vi "Edit TCP Ports.vi"(8 "error in":errorcluster) -> (0 "error out":errorcluster)   [LabVIEW 2024, in "User Interface.lvlib"]
uses:
  User Interface.lvlib
  Support/General Type Defs/Edit Devices States.ctl
  <vilib>/Utility/miscctls.llb/LVRowAndColumnTypeDef.ctl
  <vilib>/Utility/error.llb/Trim Whitespace One-Sided.vi
  Support/General Type Defs/Global Data.vi
  Data Base/DataBase Queue - Enqueue.vi
  Support/General Type Defs/General Type Definitions.lvlib
  Data Base/Data Base.lvlib
panel:
  out "Port To Delete":string[](array[string])
  in  "Delete":bool
  in  "Linux TCP Ports":string[][](table)
  in  "Windows TCP Ports":string[][](table)
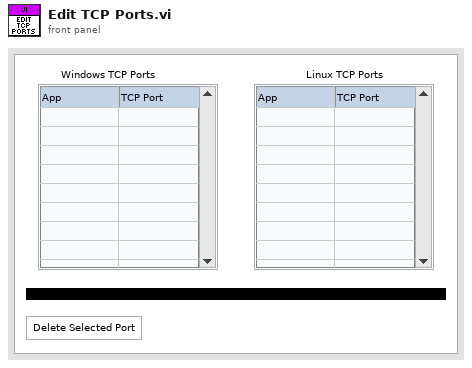
[diagram p1: front panel]
types:
  T1 = typedef "General Type Definitions.lvlib/Edit Devices States.ctl" = enum16{"Init", "IDLE", "Display Selection", "Clean Selection", "Delete", "Update", "Save Changes", "STOP"}
  T2 = typedef "LVRowAndColumnTypeDef.ctl" = cluster{"Row":i32, "Column":i32}
  T3 = enum16{"Left Button", "Center Button", "Right Button", "Window Close"}
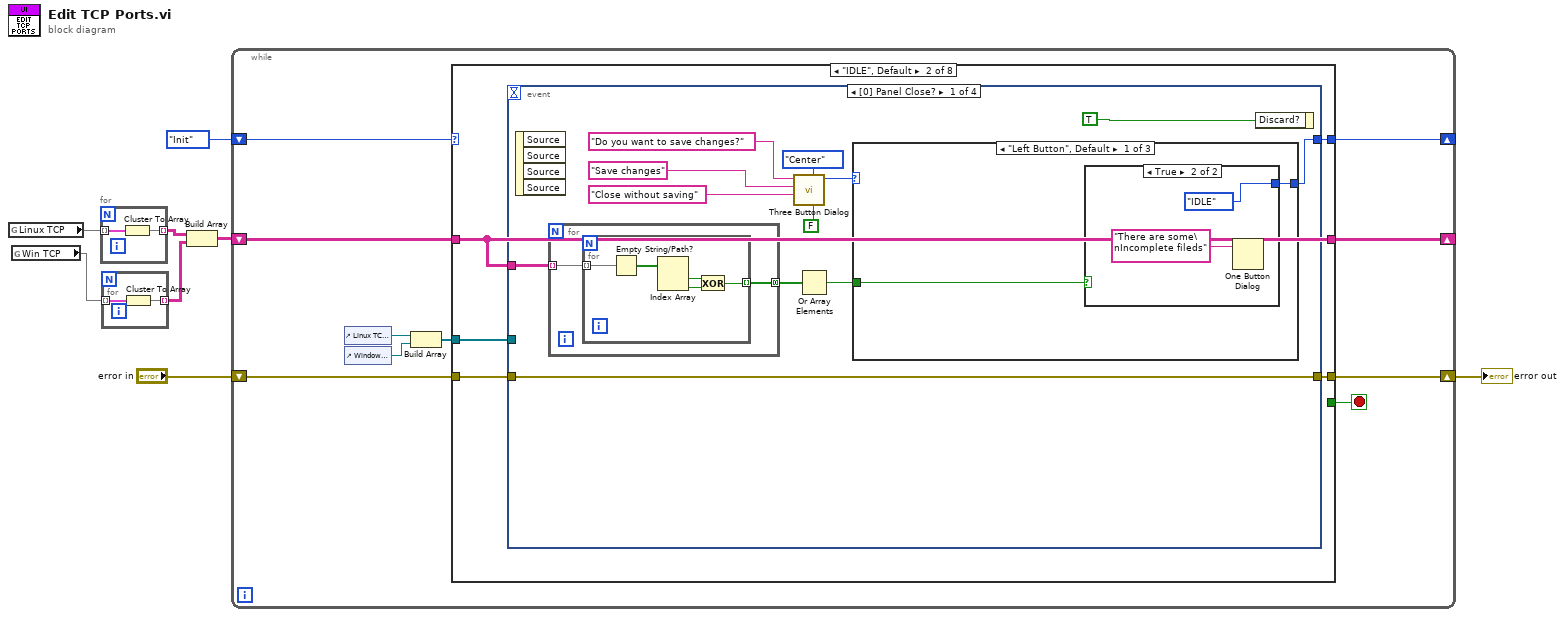
[diagram p0: block diagram]
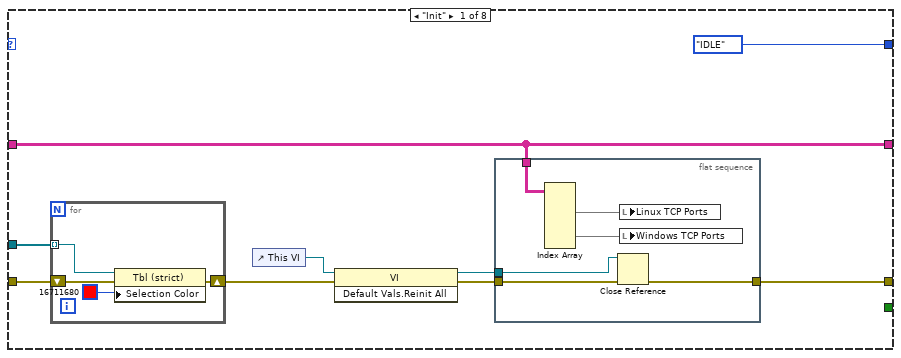
[diagram p2: hidden frame]
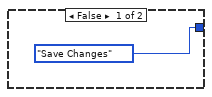
[diagram p3: hidden frame]
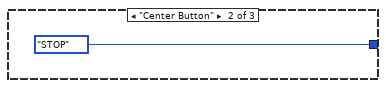
[diagram p4: hidden frame]
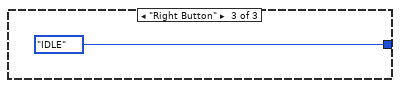
[diagram p5: hidden frame]
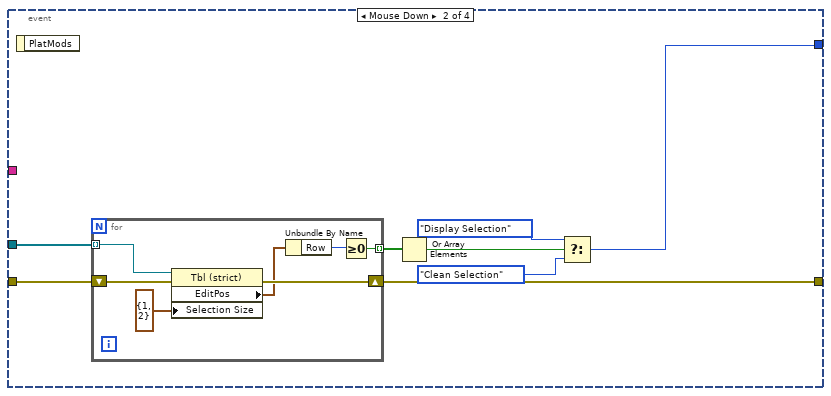
[diagram p6: hidden frame]
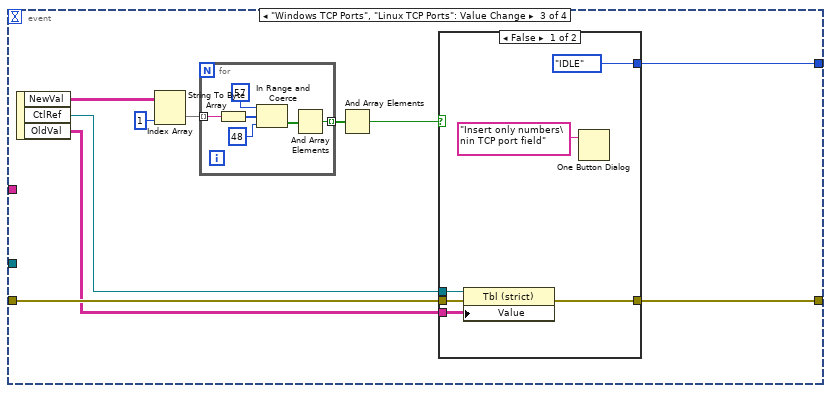
[diagram p7: hidden frame]
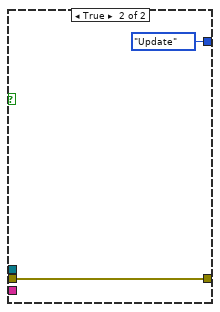
[diagram p8: hidden frame]
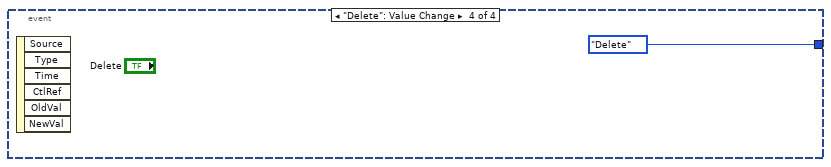
[diagram p9: hidden frame]
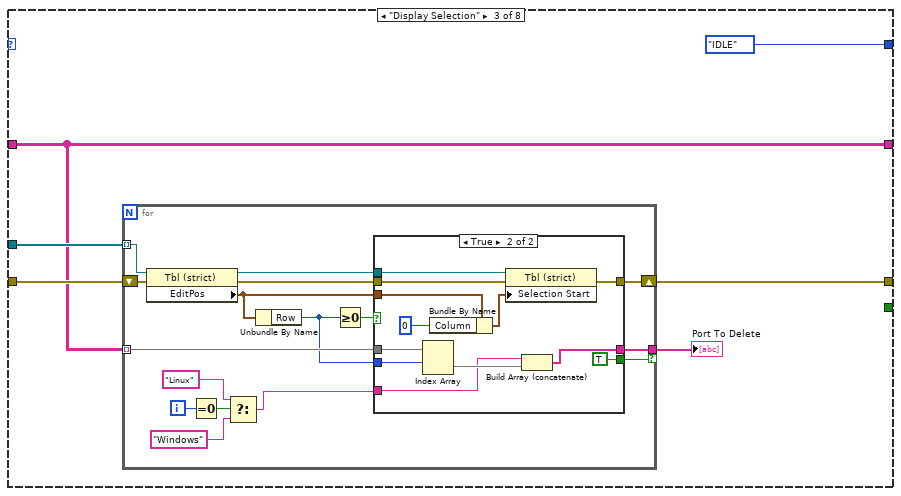
[diagram p10: hidden frame]
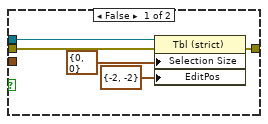
[diagram p11: hidden frame]
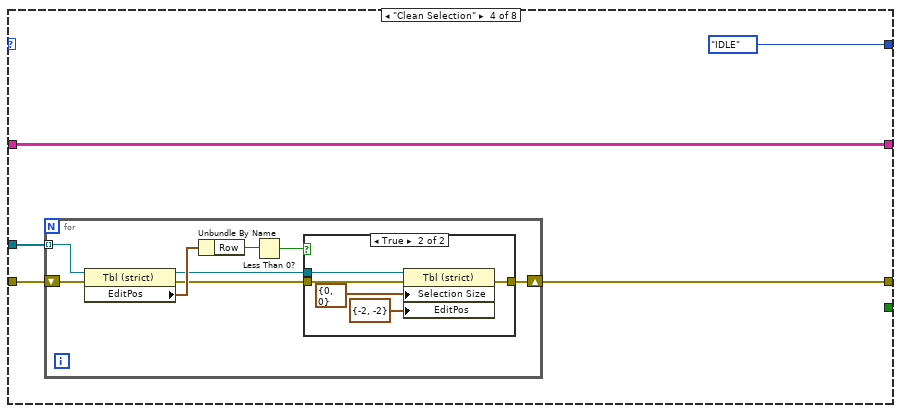
[diagram p12: hidden frame]
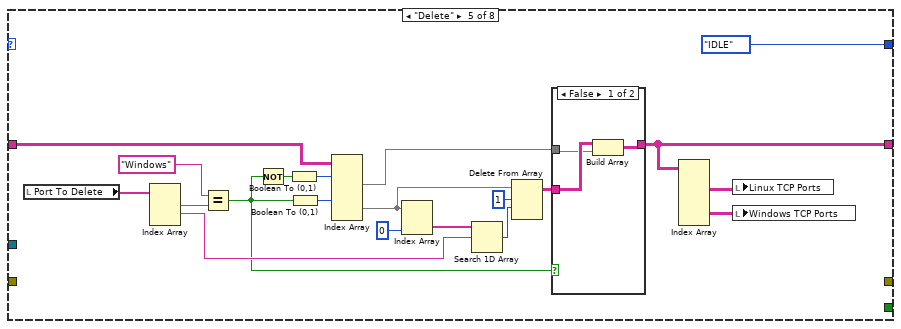
[diagram p14: hidden frame]
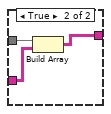
[diagram p15: hidden frame]
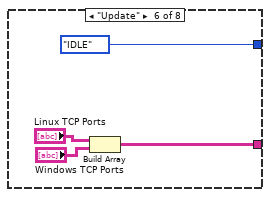
[diagram p16: hidden frame]
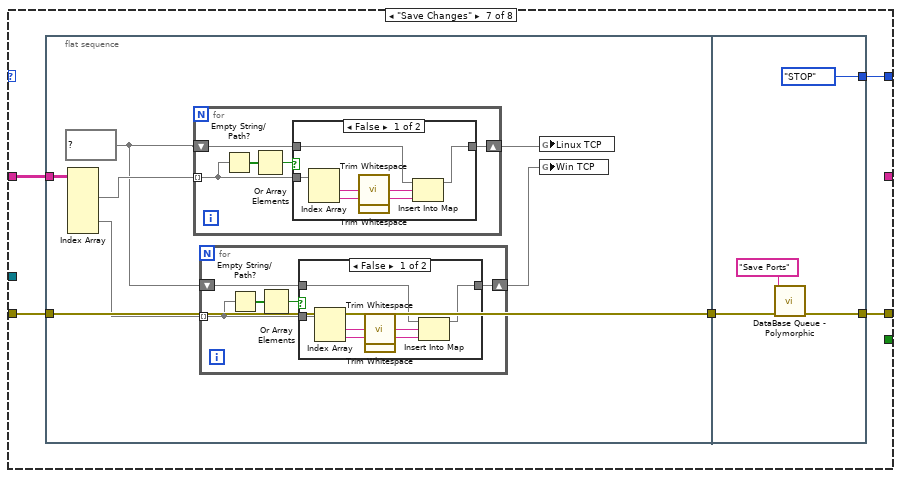
[diagram p17: hidden frame]
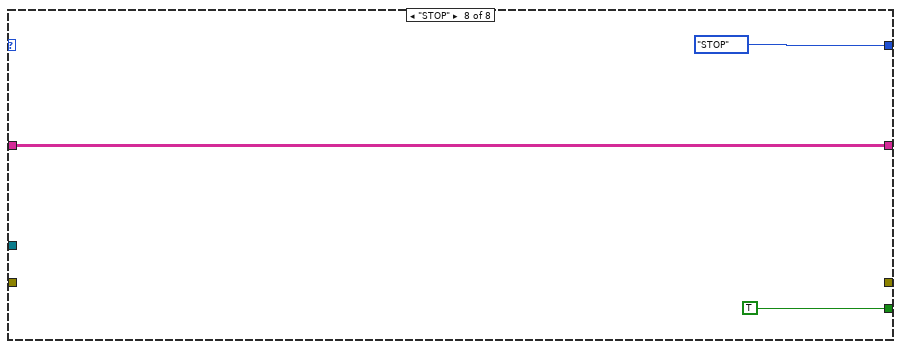
[diagram p20: hidden frame]
diagram:
  n1 = global read "Global Data.vi" "Linux TCP"() -> (w7:map{string, string})
  n2 = global read "Global Data.vi" "Win TCP"() -> (w2:map{string, string})
  n3 = for {
    tunnel: w7 -> [w10] mode=indexing
    tunnel: [w9] -> w5 mode=indexing
    n4 = Cluster To Array(cluster=w10) -> (array=w9:string[])
  }
  n5 = for {
    tunnel: [w12] -> w1 mode=indexing
    tunnel: w2 -> [w11] mode=indexing
    n6 = Cluster To Array(cluster=w11) -> (array=w12:string[])
  }
  n7 = Build Array(w5, w1) -> (w4:string[][][])
  n8 = while {
    shift-right: [w21] -> _
    shift-left: Edit_Devices_States."Init" ("Enum") -> [w22]
    shift-right: [w13] -> _
    shift-left: w4 -> [w16]
    shift-right: [w18] -> w3
    shift-left: "error in" -> [w19]
    stop <- w20 stop-if-true
    n9 = control-ref of="Linux TCP Ports"() -> (w15:refnum<vi>)
    n10 = control-ref of="Windows TCP Ports"() -> (w14:refnum<vi>)
    n11 = Build Array(w15, w14) -> (w17:refnum<vi>[])
    n12 = case shown="\"IDLE\", Default" w22 {
      tunnel: w16 -> [w23 w42 w114 w156 w183 _ w205 w245]
      tunnel: [w23 w42 w114 w156 w173 w198 _ w245] -> w13
      tunnel: [Edit_Devices_States."IDLE" ("Enum") w46 Edit_Devices_States."IDLE" Edit_Devices_States."IDLE" Edit_Devices_States."IDLE" Edit_Devices_States."IDLE" w201 Edit_Devices_States."STOP"] -> w21
      tunnel: [_ _ _ _ _ _ _ TRUE] -> w20
      tunnel: w19 -> [w30 w45 w117 w155 _ _ w204 _]
      tunnel: [w25 w44 w116 w153 _ _ w202 _] -> w18
      tunnel: w17 -> [w24 w43 w118 w154 _ _ _ _]
      frame "Init" {
        n13 = for {
          tunnel: w24 -> [w41] mode=indexing
          shift-right: [w40] -> w26
          shift-left: w30 -> [w39]
          n14 = property class="Tbl (strict)"(reference=w41, error in=w39, "Selection Color"=u32 16711680) -> (error out=w40:errorcluster)  [unwired: 1 out]
        }
        n15 = control-ref of="This VI"() -> (w27:refnum<vi>)
        n16 = invoke class="VI" method="Default Vals.Reinit All"(reference=w27, error in=w26) -> (reference out=w29:refnum<vi>, error out=w28:errorcluster)  [unwired: 1 in, 1 out]
        n17 = flat-sequence {
          tunnel: w29 -> [w37]
          tunnel: w28 -> [w36]
          tunnel: [w35] -> w25
          tunnel: w23 -> [w34]
          frame #0 {
            n18 = Index Array(array=w34) -> (element #1=w33:string[][], element #2=w32:string[][])  [unwired: 6 in]
            n19 = Close Reference(reference=w37, error in (no error)=w36) -> (error out=w35:errorcluster)
            n20 = local write "Linux TCP Ports"(w33) -> ()
            n21 = local write "Windows TCP Ports"(w32) -> ()
          }
        }
      }
      frame "IDLE", Default {
        n22 = event shown="[0] Panel Close?" {
          selector: _ -> [_ _ _ _]
          dyn-events: _ -> [_ _ _ _]
          timeout: _ -> [_ _ _ _]
          tunnel: [w51 w73 w95 Edit_Devices_States."Delete"] -> w46
          tunnel: w45 -> [w50 w79 w91 _]
          tunnel: [w50 w77 w89 _] -> w44
          tunnel: w43 -> [_ w80 _ _]
          tunnel: w42 -> [w49 _ _ _]
          event Panel Close? {
            n23 = event-data() -> ()  [unwired: 1 in, 4 out]
            n24 = for {
              tunnel: w49 -> [w60] mode=indexing
              tunnel: [w59] -> w48 mode=concatenating
              n25 = for {
                tunnel: w60 -> [w65] mode=indexing
                tunnel: [w61] -> w59 mode=indexing
                n26 = Empty String/Path?(string/path=w65) -> (empty?=w64:bool[])
                n27 = Index Array(array=w64) -> (element #1=w63:bool, element #2=w62:bool)  [unwired: 2 in]
                n28 = Exclusive Or(1:w62, 2:w63) -> (0:w61:bool)
              }
            }
            n29 = call <vilib>:"Three Button Dialog.vi"("Allow user to close window? (TRUE)"=FALSE, "Justify Message (Left)"=enum16{"Left", "Center", "Right"}."Center", "Center Button Text (\"No\")"="Close without saving" ("Center Button Text (\"No\")"), "Left Button Text (\"Yes\")"="Save changes" ("Left Button Text (\"Yes\")"), "message"="Do you want to save changes?") -> ("Which Button?"=w55:T3)  [unwired: 6 in]
            n30 = Or Array Elements(Boolean array=w48) -> (logical OR=w47:bool)
            n31 = case shown="\"Left Button\", Default" w55 {
              tunnel: [w67 Edit_Devices_States."STOP" Edit_Devices_States."IDLE"] -> w51
              tunnel: w47 -> [w66 _ _]
              frame "Left Button", Default {
                n32 = case shown="True" w66 {
                  tunnel: [Edit_Devices_States."Save Changes" Edit_Devices_States."IDLE"] -> w67
                  frame False {
                  }
                  frame True {
                    n33 = One Button Dialog(message="There are some\nIncomplete fileds") -> ()  [unwired: 1 in, 1 out]
                  }
                }
              }
              frame "Center Button" {
              }
              frame "Right Button" {
              }
            }
            n34 = event-data("Discard?"=TRUE) -> ()  [unwired: 1 in, 1 out]
          }
          event Mouse Down {
            n35 = event-data() -> ()  [unwired: 1 in, 1 out]
            n36 = for {
              tunnel: w80 -> [w87] mode=indexing
              shift-right: [w85] -> w77
              shift-left: w79 -> [w86]
              tunnel: [w81] -> w78 mode=indexing
              n37 = property class="Tbl (strict)"(reference=w87, error in=w86, "Selection Size"=T2 {"Row"=1, "Column"=2}) -> (error out=w85:errorcluster, "EditPos"=w83:T2)  [unwired: 1 out]
              n38 = Unbundle By Name(w83) -> ("Row"=w82:i32)
              n39 = Greater Or Equal To 0?(x=w82) -> (x >= 0?=w81:bool)
            }
            n40 = Or Array Elements(Boolean array=w78) -> (logical OR=w74:bool)
            n41 = Select(t=Edit_Devices_States."Display Selection", s=w74, f=Edit_Devices_States."Clean Selection") -> (s? t:f=w73:T1)
          }
          event "Windows TCP Ports", "Linux TCP Ports": Value Change {
            n42 = event-data() -> ("NewVal"=w88:string[][], "CtlRef"=w92:refnum<vi>, "OldVal"=w90:string[][])  [unwired: 1 in]
            n43 = Index Array(array=w88, index (col)=1) -> (element=w94:string[])  [unwired: 1 in]
            n44 = for {
              tunnel: w94 -> [w101] mode=indexing
              tunnel: [w98] -> w93 mode=indexing
              n45 = String To Byte Array(string=w101) -> (unsigned byte array=w100:u8[])
              n46 = In Range and Coerce(upper limit=57, x=w100, lower limit=48) -> (In Range?=w99:bool[])  [unwired: 1 out]
              n47 = And Array Elements(Boolean array=w99) -> (logical AND=w98:bool)
            }
            n48 = And Array Elements(Boolean array=w93) -> (logical AND=w96:bool)
            n49 = case shown="False" w96 {
              tunnel: [Edit_Devices_States."IDLE" Edit_Devices_States."Update"] -> w95
              tunnel: w92 -> [w107 _]
              tunnel: w91 -> [w106 w110]
              tunnel: w90 -> [w105 _]
              tunnel: [w104 w110] -> w89
              frame False {
                n50 = property class="Tbl (strict)"(reference=w107, error in=w106, "Value"=w105) -> (error out=w104:errorcluster)  [unwired: 1 out]
                n51 = One Button Dialog(message="Insert only numbers\nin TCP port field") -> ()  [unwired: 1 in, 1 out]
              }
              frame True {
              }
            }
          }
          event "Delete": Value Change {
            n52 = event-data() -> ()  [unwired: 1 in, 6 out]
          }
        }
      }
      frame "Display Selection" {
        n53 = for {
          tunnel: w118 -> [w134] mode=indexing
          shift-right: [w132] -> w116
          shift-left: w117 -> [w133]
          tunnel: w114 -> [w127] mode=indexing
          tunnel: [w119] -> w113 if=w125
          i -> [w124]
          n54 = property class="Tbl (strict)"(reference=w134, error in=w133) -> (reference out=w130:refnum<vi>, error out=w131:errorcluster, "EditPos"=w129:T2)
          n55 = Equal To 0?(x=w124) -> (x = 0?=w123:bool)
          n56 = Select(t="Linux", s=w123, f="Windows") -> (s? t:f=w120:string)
          n57 = Unbundle By Name(w129) -> ("Row"=w126:i32)
          n58 = Greater Or Equal To 0?(x=w126) -> (x >= 0?=w128:bool)
          n59 = case shown="True" w128 {
            tunnel: [w137 w151] -> w132
            tunnel: w131 -> [w136 w150]
            tunnel: w130 -> [w135 w149]
            tunnel: w129 -> [_ w148]
            tunnel: w127 -> [_ w145]
            tunnel: w126 -> [_ w144]
            tunnel: [_ TRUE] -> w125
            tunnel: w120 -> [_ w141]
            tunnel: [_ w140] -> w119
            frame False {
              n60 = property class="Tbl (strict)"(reference=w135, error in=w136, "Selection Size"=T2 {"Row"=0, "Column"=0}, "EditPos"=T2 {"Row"=-2, "Column"=-2}) -> (error out=w137:errorcluster)  [unwired: 1 out]
            }
            frame True {
              n61 = Index Array(array=w145, index (row)=w144) -> (element=w142:string[])  [unwired: 1 in]
              n62 = Bundle By Name(cluster=w148, "Column"=0) -> (w146:T2)
              n63 = property class="Tbl (strict)"(reference=w149, error in=w150, "Selection Start"=w146) -> (error out=w151:errorcluster)  [unwired: 1 out]
              n64 = Build Array (concatenate)(w141, w142) -> (w140:string[])
            }
          }
        }
        "Port To Delete" <- w113
      }
      frame "Clean Selection" {
        n65 = for {
          tunnel: w154 -> [w164] mode=indexing
          shift-right: [w160] -> w153
          shift-left: w155 -> [w163]
          n66 = property class="Tbl (strict)"(reference=w164, error in=w163) -> (reference out=w158:refnum<vi>, error out=w159:errorcluster, "EditPos"=w162:T2)
          n67 = Unbundle By Name(w162) -> ("Row"=w161:i32)
          n68 = Less Than 0?(x=w161) -> (x < 0?=w157:bool)
          n69 = case shown="True" w157 {
            tunnel: [w165 w168] -> w160
            tunnel: w159 -> [w165 w167]
            tunnel: w158 -> [_ w166]
            frame False {
            }
            frame True {
              n70 = property class="Tbl (strict)"(reference=w166, error in=w167, "Selection Size"=T2 {"Row"=0, "Column"=0}, "EditPos"=T2 {"Row"=-2, "Column"=-2}) -> (error out=w168:errorcluster)  [unwired: 1 out]
            }
          }
        }
      }
      frame "Delete" {
        n71 = local read "Port To Delete"() -> (w189:string[])
        n72 = Index Array(array=w189) -> (element #1=w188:string, element #2=w184:string)  [unwired: 3 in, 1 out]
        n73 = Equal?(x="Windows" ("element"), y=w188) -> (x = y?=w176:bool)
        n74 = Not(x=w176) -> (.not. x?=w180:bool)
        n75 = Boolean To (0,1)(Boolean=w180) -> (0, 1=w181:i16)
        n76 = Boolean To (0,1)(Boolean=w176) -> (0, 1=w182:i16)
        n77 = Index Array(array=w183, index (dim 0) #1=w181, index (dim 0) #2=w182) -> (element #1=w175:string[][], element #2=w179:string[][])  [unwired: 4 in]
        n78 = Index Array(array=w179, index (col)=0) -> (element=w185:string[])  [unwired: 1 in]
        n79 = Search 1D Array(1D array=w185, element=w184) -> (index of element=w177:i32)  [unwired: 1 in]
        n80 = Delete From Array(array=w179, length=1, index (row)=w177) -> (array with subset deleted=w174:string[][])  [unwired: 1 in, 1 out]
        n81 = case shown="False" w176 {
          tunnel: w175 -> [w192 w196]
          tunnel: w174 -> [w193 w195]
          tunnel: [w191 w194] -> w173
          frame False {
            n82 = Build Array(w193, w192) -> (w191:string[][][])
          }
          frame True {
            n83 = Build Array(w196, w195) -> (w194:string[][][])
          }
        }
        n84 = Index Array(array=w173) -> (element #1=w172:string[][], element #2=w171:string[][])  [unwired: 6 in]
        n85 = local write "Linux TCP Ports"(w172) -> ()
        n86 = local write "Windows TCP Ports"(w171) -> ()
      }
      frame "Update" {
        n87 = Build Array("Linux TCP Ports", "Windows TCP Ports") -> (w198:string[][][])
      }
      frame "Save Changes" {
        n88 = flat-sequence {
          tunnel: w205 -> [w211]
          tunnel: w204 -> [w212]
          tunnel: [w212] -> w203
          tunnel: w203 -> [w241]
          tunnel: [w240] -> w202
          tunnel: [Edit_Devices_States."STOP"] -> w201
          frame #0 {
            w206 = map{string, string} {} ("map")
            n89 = Index Array(array=w211) -> (element #1=w207:string[][], element #2=w210:string[][])  [unwired: 6 in]
            n90 = for {
              shift-right: [w217] -> w208
              shift-left: w206 -> [w216]
              tunnel: w207 -> [w214] mode=indexing
              n91 = Empty String/Path?(string/path=w214) -> (empty?=w215:bool[])
              n92 = Or Array Elements(Boolean array=w215) -> (logical OR=w213:bool)
              n93 = case shown="False" w213 {
                tunnel: [w224 w225] -> w217
                tunnel: w216 -> [w223 w225]
                tunnel: w214 -> [w222 _]
                frame False {
                  n94 = Index Array(array=w222) -> (element #1=w221:string, element #2=w220:string)  [unwired: 2 in]
                  n95 = call <vilib>:"Trim Whitespace.vi"("string"=w221) -> ("trimmed string"=w219:string)  [unwired: 1 in]
                  n96 = call <vilib>:"Trim Whitespace.vi"("string"=w220) -> ("trimmed string"=w218:string)  [unwired: 1 in]
                  n97 = Insert Into Map(map in=w223, key=w219, value=w218) -> (map out=w224:map{string, string})  [unwired: 2 out]
                }
                frame True {
                }
              }
            }
            n98 = for {
              shift-right: [w230] -> w209
              shift-left: w206 -> [w229]
              tunnel: w210 -> [w227] mode=indexing
              n99 = Empty String/Path?(string/path=w227) -> (empty?=w228:bool[])
              n100 = Or Array Elements(Boolean array=w228) -> (logical OR=w226:bool)
              n101 = case shown="False" w226 {
                tunnel: [w237 w238] -> w230
                tunnel: w229 -> [w236 w238]
                tunnel: w227 -> [w235 _]
                frame False {
                  n102 = Index Array(array=w235) -> (element #1=w234:string, element #2=w233:string)  [unwired: 2 in]
                  n103 = call <vilib>:"Trim Whitespace.vi"("string"=w234) -> ("trimmed string"=w232:string)  [unwired: 1 in]
                  n104 = call <vilib>:"Trim Whitespace.vi"("string"=w233) -> ("trimmed string"=w231:string)  [unwired: 1 in]
                  n105 = Insert Into Map(map in=w236, key=w232, value=w231) -> (map out=w237:map{string, string})  [unwired: 2 out]
                }
                frame True {
                }
              }
            }
            n106 = global write "Global Data.vi" "Linux TCP"(w208) -> ()
            n107 = global write "Global Data.vi" "Win TCP"(w209) -> ()
          }
          frame #1 {
            n108 = call-poly "DataBase Queue - Polymorphic.vi"("error in"=w241, "Message"="Save Ports") -> ("error out"=w240:errorcluster)  [unwired: 9 in]
          }
        }
      }
      frame "STOP" {
      }
    }
  }
  "error out" <- w3
